vi "Teleop[Conflict 1].vi"(10 "Match Info":T3={"Autonomous Elapsed Seconds"=0.0, "TeleOp Elapsed Seconds"=0.0, "Disabled Elapsed Seconds"=0.0, "Visited Autonomous"=FALSE, "Visited TeleOp"=FALSE, "Visited Disabled"=FALSE, "Autonomous Settings"={"Autonomous Style"=enum."Independent", "VI Refnum"=refnum}}, 11 "Call Context":T4) -> ()   [LabVIEW 2019]
doc: "This VI is called for each TeleOp packet received from the DS where the robot is not disabled. It is often used to read from the joysticks and update I/O or to update setpoints for timed control loops. It should complete and return within 20 milliseconds or it may miss DS packets."
uses:
  <vilib>/Rock Robotics/WPI/DriverStation/WPI_DriverStationDerivedRobotMode.ctl
  <vilib>/Rock Robotics/WPI/DriverStation/WPI_DriverStationMatch Info.ctl
  <vilib>/Rock Robotics/WPI/ThirdParty/Phoenix-LabVIEW/Motor Controller/Controls/CTRE_Phoenix_MotorControl_ControlMode.ctl
  <vilib>/Rock Robotics/WPI/Utilities/WPI_GetSetVariantRefNum.vi
  <vilib>/Rock Robotics/WPI/Joystick/WPI_JoystickArcadeMapping.vi
  Toolbox/Piston/Piston Toggle.vi
  <vilib>/Rock Robotics/WPI/Solenoid/WPI_SolenoidSetEnum.vi
  <vilib>/Rock Robotics/Network Tables/NT Write Number.vi
  <vilib>/Rock Robotics/Network Tables/NT Read Number.vi
  <vilib>/addons/control/pid/pid.llb/PID (DBL).vi
  <vilib>/Rock Robotics/WPI/ThirdParty/Phoenix-LabVIEW/Motor Controller/Get/CTRE_Phoenix_MotorController_GetSupplyAndStatorCurrent_Enhanced.vi
  <vilib>/addons/control/pid/NI_PID_pid.lvlib
panel:
  in  "Magazine Power":dbl=0.25
  in  "Shooter Power":dbl=1.0
  in  "Magazine Overflow Power":dbl=-1.0
  in  "Magazine Intake Power":dbl=0.25
  in  "Intake power":dbl=0.7
  out "Shooter Motor Current":T1(graph)
  out "tx":dbl
  in  "PID gains":T2={"proportional gain (Kc)"=0.025, "integral time (Ti, min)"=0.01, "derivative time (Td, min)"=0.0} {"derivative time (Td, min)" format="%.3g"; "integral time (Ti, min)" format="%.3e"; "proportional gain (Kc)" format="%.3g"}
  in  "Winch Power":dbl=1.0
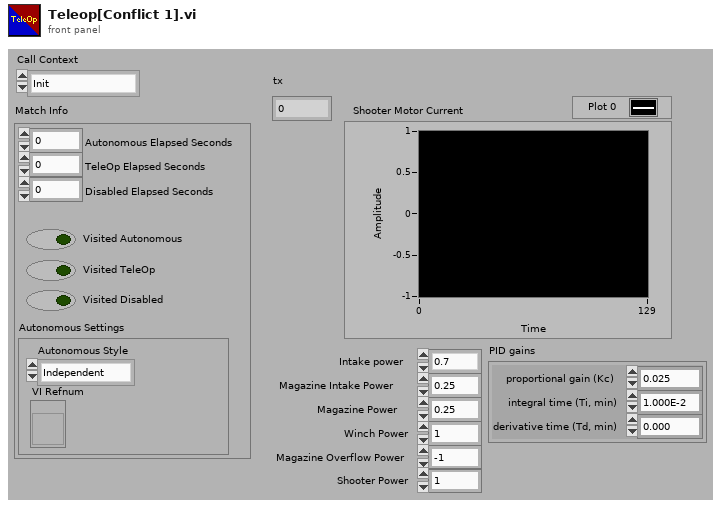
[diagram p1: front panel]
types:
  T1 = cluster{"Supply Current":dbl, "Stator Current":dbl}
  T2 = cluster{"proportional gain (Kc)":dbl, "integral time (Ti, min)":dbl, "derivative time (Td, min)":dbl}
  T3 = typedef "WPI_DriverStationMatch Info.ctl" = cluster{"Autonomous Elapsed Seconds":dbl, "TeleOp Elapsed Seconds":dbl, "Disabled Elapsed Seconds":dbl, "Visited Autonomous":bool, "Visited TeleOp":bool, "Visited Disabled":bool, "Autonomous Settings":cluster{"Autonomous Style":enum16{"Iterative", "Independent"}, "VI Refnum":refnum<vi>}}
  T4 = typedef "WPI_DriverStationDerivedRobotMode.ctl" = enum16{"Init", "Execute", "Stop"}
  T5 = typedef "CTRE_Phoenix_MotorControl_ControlMode.ctl" = u16
  T6 = cluster{"Intake In":bool, "Intake Out":bool, "Magazine In":bool, "Magazine Out":bool, "Winch In":bool, "Winch Out":bool, "Climber Hold":bool, "Intake Pistons":bool, "Shooter Hold":bool, "None":bool, "Power Toggle":bool, "Auto Target":bool}
  T7 = typedef "WPI_JoystickDevRef.ctl" = cluster{"Device":T8}
  T8 = typedef "WPI_JoystickDeviceEnum.ctl" = enum16{"USB 0", "USB 1", "USB 2", "USB 3", "USB 4", "USB 5"}
  T9 = typedef "WPI_MotorControlDeviceRef.ctl" = cluster{"DeviceStatus":errorcluster, "Type":T10, "PWM":cluster{"PWM Channel":T11, "DeadBand":T12}, "CAN":cluster{"Device Number":u8, "SetOutput VI Ref":variant, "GetOutput VI Ref":variant, "Enable VI Ref":variant, "Disable VI Ref":variant, "Data":variant}, "Invert":bool, "DIO PWM":cluster{"PWM \"Enable\" Channel":T11, "DIOChannel":T13, "PWM Rate":dbl}}
  T10 = typedef "WPI_MotorControlType.ctl" = enum16{"PWM", "CAN", "DIO PWM"}
  T11 = typedef "FPGA_DIOPWMChannel.ctl" = enum8{"PWM 0", "PWM 1", "PWM 2", "PWM 3", "PWM 4", "PWM 5", "PWM 6", "PWM 7", "PWM 8", "PWM 9", "PWM MXP 0", "PWM MXP 1", "PWM MXP 2", "PWM MXP 3", "PWM MXP 4", "PWM MXP 5", "PWM MXP 6", "PWM MXP 7", "PWM MXP 8", "PWM MXP 9", "Invalid"}
  T12 = typedef "WPI_PWMDeadband.ctl" = cluster{"Name":string, "maxPositivePwm":i32, "minPositivePwm":i32, "centerPwm":i32, "maxNegativePwm":i32, "minNegativePwm":i32, "angularRange":u16}
  T13 = typedef "FPGA_DIOChannel.ctl" = enum8{"DIO 0", "DIO 1", "DIO 2", "DIO 3", "DIO 4", "DIO 5", "DIO 6", "DIO 7", "DIO 8", "DIO 9", "DIO MXP 0", "DIO MXP 1", "DIO MXP 2", "DIO MXP 3", "DIO MXP 4", "DIO MXP 5", "DIO MXP 6", "DIO MXP 7", "DIO MXP 8", "DIO MXP 9", "DIO MXP 10", "DIO MXP 11", "DIO MXP 12", "DIO MXP 13", "DIO MXP 14", "DIO MXP 15", "SPI Port CS1", "SPI Port CS2", "SPI Port CS3", "SPI Port MISO", "SPI Port MOSI", "Invalid"}
  T14 = typedef "WPI_SolenoidValue.ctl" = enum16{"Off", "On", "Forward", "Reverse"}
  T15 = typedef "WPI_SolenoidDevRef.ctl" = cluster{"DevStatus":errorcluster, "Pneumatics Control Module":u8, "Forward Solenoid Channel":T16, "Reverse Solenoid Channel":T16}
  T16 = typedef "WPI_SolenoidChannel.ctl" = enum8{"Solenoid 0", "Solenoid 1", "Solenoid 2", "Solenoid 3", "Solenoid 4", "Solenoid 5", "Solenoid 6", "Solenoid 7", "Invalid"}
  T17 = typedef "WPI_DigitalInputDevRef.ctl" = cluster{"DevStatus":errorcluster, "DIO Channel":T13}
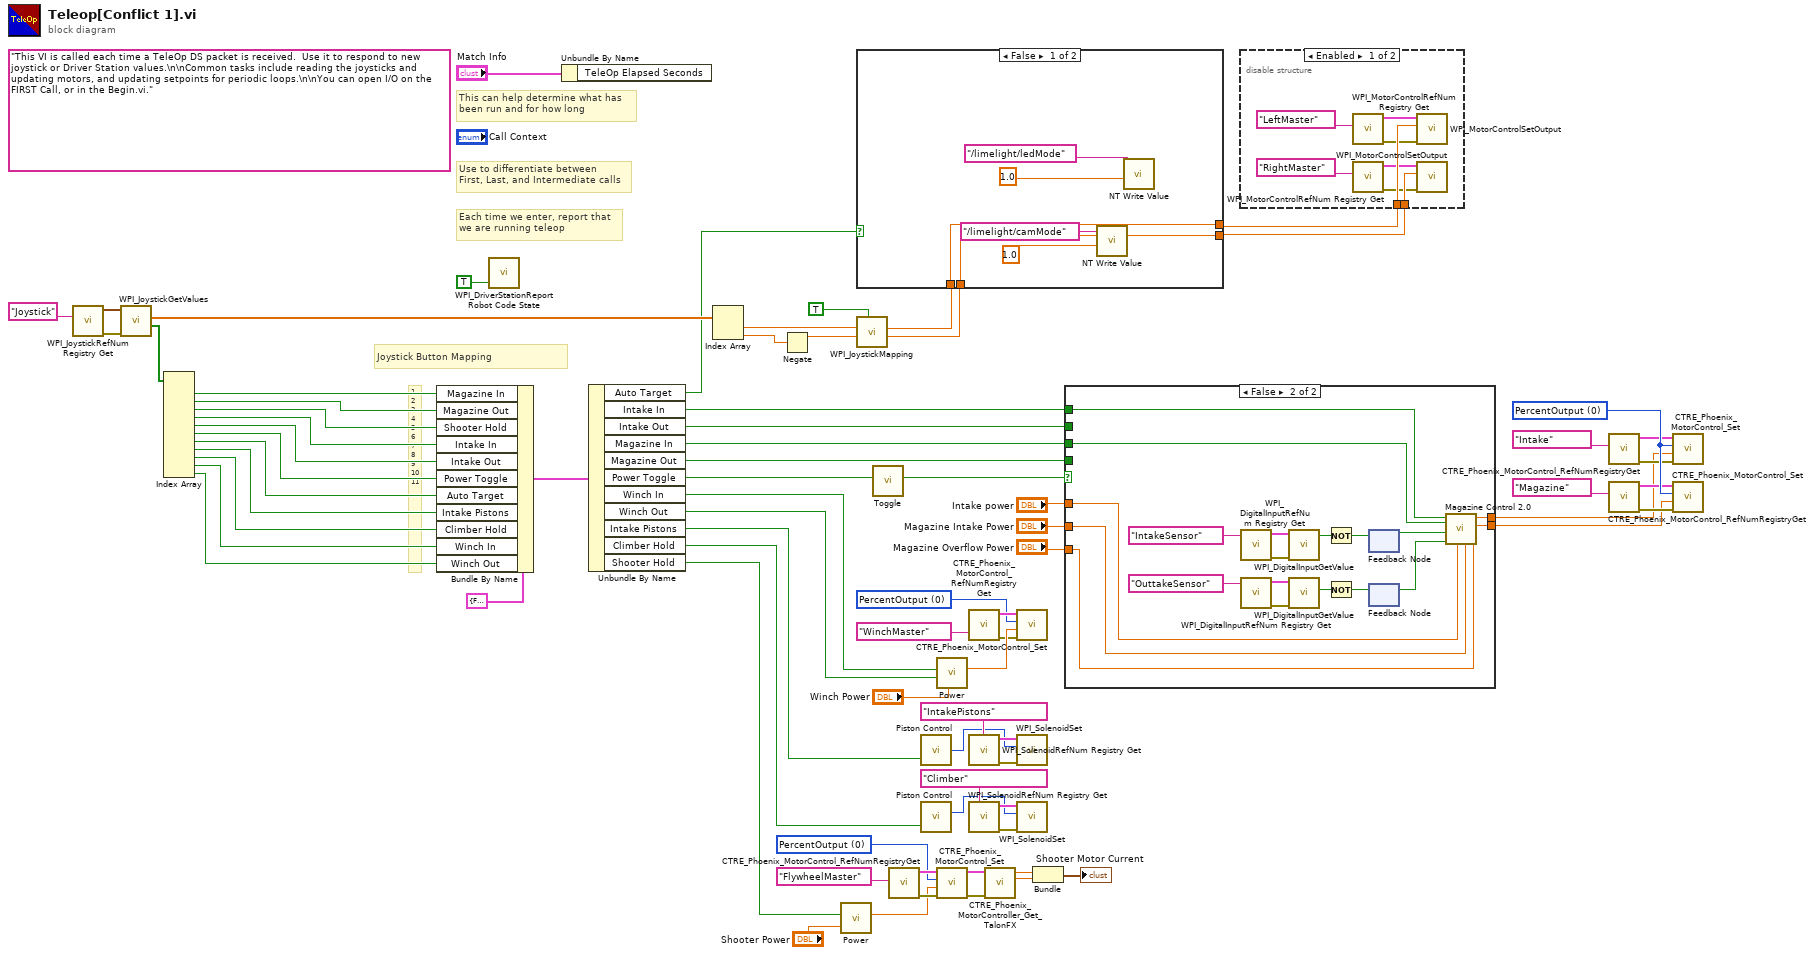
[diagram p0: block diagram]
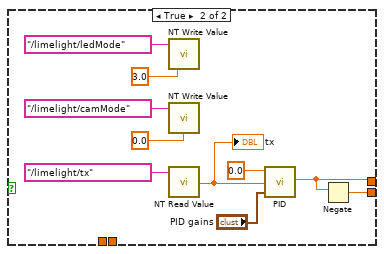
[diagram p2: hidden frame]
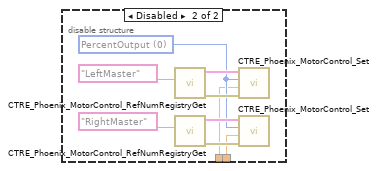
[diagram p3: hidden frame]
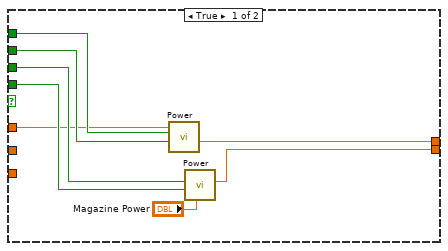
[diagram p4: hidden frame]
diagram:
  w8 = T5 0 items=["PercentOutput"=0, "Position"=1, "Velocity"=2, "Current"=3, "Follower"=5, "MotionProfile"=6, "MotionMagic"=7, "MotionProfileArc"=10, "Disabled"=15] ("Control Mode")
  w21 = T5 0 items=["PercentOutput"=0, "Position"=1, "Velocity"=2, "Current"=3, "Follower"=5, "MotionProfile"=6, "MotionMagic"=7, "MotionProfileArc"=10, "Disabled"=15] ("Control Mode")
  w25 = T5 0 items=["PercentOutput"=0, "Position"=1, "Velocity"=2, "Current"=3, "Follower"=5, "MotionProfile"=6, "MotionMagic"=7, "MotionProfileArc"=10, "Disabled"=15] ("Control Mode")
  (unwired) "This VI is called each time a TeleOp DS packet is received.  Use it to respond to new joystick or Driver Station values.\n\nCommon tasks include reading the joysticks and updating motors, and updating setpoints for periodic loops.\n\nYou can open I/O on the FIRST Call, or in the Begin.vi."
  # "1\n2\n3\n4\n5\n6\n7\n8\n9\n10\n11"
  # "Joystick Button Mapping"
  # "Each time we enter, report that\nwe are running teleop"
  # "Use to differentiate between\nFirst, Last, and Intermediate calls"
  # "This can help determine what has\nbeen run and for how long"
  n1 = call <vilib>:"WPI_JoystickRefNum Registry Get.vi"("refnum name"="Joystick") -> ("error out"=w75:errorcluster, "JoystickDevRef"=w74:T7)  [unwired: 9 in]
  n2 = call <vilib>:"WPI_JoystickGetValues.vi"("error in (no error)"=w75, "JoystickDevRef"=w74) -> ("Buttons"=w57:bool[], "Axes"=w72:dbl[])  [unwired: 5 in, 3 out]
  n3 = Index Array(array=w57) -> (element #1=w58:bool, element #2=w29:bool, element #3=w66:bool, element #4=w30:bool, element #5=w65:bool, element #6=w64:bool, element #7=w63:bool, element #8=w62:bool, element #9=w61:bool, element #10=w60:bool, element #11=w59:bool)  [unwired: 11 in]
  n4 = Bundle By Name(cluster=T6 {"Intake In"=FALSE, "Intake Out"=FALSE, "Magazine In"=FALSE, "Magazine Out"=FALSE, "Winch In"=FALSE, "Winch Out"=FALSE, "Climber Hold"=FALSE, "Intake Pistons"=FALSE, "Shooter Hold"=FALSE, "None"=FALSE, "Power Toggle"=FALSE, "Auto Target"=FALSE} ("input cluster"), "Magazine In"=w58, "Magazine Out"=w29, "Shooter Hold"=w66, "Intake In"=w30, "Intake Out"=w65, "Power Toggle"=w64, "Auto Target"=w63, "Intake Pistons"=w62, "Climber Hold"=w61, "Winch In"=w60, "Winch Out"=w59) -> (w56:T6)
  n5 = call <vilib>:"WPI_DriverStationReport Robot Code State.vi"("TeleOp"=TRUE ("Autonomous")) -> ()  [unwired: 10 in, 1 out]
  n6 = Unbundle By Name("Match Info") -> ()  [unwired: 1 out]
  n7 = Unbundle By Name(w56) -> ("Auto Target"=w39:bool, "Intake In"=w44:bool, "Intake Out"=w55:bool, "Magazine In"=w54:bool, "Magazine Out"=w53:bool, "Power Toggle"=w23:bool, "Winch In"=w52:bool, "Winch Out"=w51:bool, "Intake Pistons"=w36:bool, "Climber Hold"=w35:bool, "Shooter Hold"=w12:bool)
  n8 = Index Array(array=w72) -> (element #1=w71:dbl, element #2=w69:dbl)  [unwired: 2 in]
  n9 = Negate(x=w69) -> (-x=w70:dbl)
  n10 = call "Power.vi"("Positive Power"="Shooter Power", "Positive"=w12) -> ("Output"=w2:dbl)  [unwired: 9 in]
  n11 = call-poly <vilib>:"WPI_JoystickMapping.vi"("Square Inputs"=TRUE, "Y axis value"=w70, "X axis value"=w71) -> ("Right Motor Value"=w42:dbl, "Left Motor Value"=w43:dbl)  [unwired: 7 in]
  n12 = case shown="False" w39 {
    tunnel: w43 -> [w83 _]
    tunnel: w42 -> [w82 _]
    tunnel: [w83 w88] -> w41
    tunnel: [w82 w89] -> w40
    frame False {
      n13 = call-poly <vilib>:"NT Write Value.vi"("Numeric"=1.0, "Name"="/limelight/camMode") -> ()  [unwired: 9 in, 1 out]
      n14 = call-poly <vilib>:"NT Write Value.vi"("Numeric"=1.0, "Name"="/limelight/ledMode") -> ()  [unwired: 9 in, 1 out]
    }
    frame True {
      n15 = call-poly <vilib>:"NT Write Value.vi"("Numeric"=3.0, "Name"="/limelight/ledMode") -> ()  [unwired: 9 in, 1 out]
      n16 = call-poly <vilib>:"NT Write Value.vi"("Numeric"=0.0, "Name"="/limelight/camMode") -> ()  [unwired: 9 in, 1 out]
      n17 = call-poly <vilib>:"NT Read Value.vi"("Name"="/limelight/tx") -> ("Numeric"=w92:dbl)  [unwired: 9 in, 1 out]
      "tx" <- w92
      n18 = call-poly <vilib>:"PID.vi"("PID gains"="PID gains", "process variable"=w92, "setpoint"=0.0) -> ("output"=w88:dbl)  [unwired: 7 in, 1 out]
      n19 = Negate(x=w88) -> (-x=w89:dbl)
    }
  }
  n20 = call "Toggle.vi"("Input"=w23) -> ("Output"=w24:bool)  [unwired: 10 in]
  n21 = call <vilib>:"CTRE_Phoenix_MotorControl_RefNumRegistryGet.vi"("refnum name"="FlywheelMaster") -> ("error out"=w10:errorcluster, "PhoenixMotorControlDevRef"=w9:T9)  [unwired: 9 in]
  n22 = call-poly "Piston Control.vi"("Input"=w36) -> ("Output"=w38:T14)  [unwired: 1 in]
  n23 = call-poly "Piston Control.vi"("Input"=w35) -> ("Output"=w37:T14)  [unwired: 1 in]
  n24 = call "Power.vi"("Positive Power"="Winch Power", "Negative"=w51, "Positive"=w52) -> ("Output"=w67:dbl)  [unwired: 8 in]
  n25 = call <vilib>:"CTRE_Phoenix_MotorControl_Set.vi"("error in (no error)"=w10, "Output"=w2, "Control Mode"=w8, "PhoenixMotorControlDevRef"=w9) -> ("error out"=w6:errorcluster, "PhoenixMotorControlDevRef"=w7:T9)  [unwired: 6 in]
  n26 = call <vilib>:"CTRE_Phoenix_MotorControl_RefNumRegistryGet.vi"("refnum name"="WinchMaster") -> ("error out"=w27:errorcluster, "PhoenixMotorControlDevRef"=w26:T9)  [unwired: 9 in]
  n27 = call <vilib>:"WPI_SolenoidRefNum Registry Get.vi"("refnum name"="IntakePistons") -> ("error out"=w50:errorcluster, "SolenoidDevRef"=w49:T15)  [unwired: 9 in]
  n28 = call <vilib>:"WPI_SolenoidRefNum Registry Get.vi"("refnum name"="Climber") -> ("error out"=w47:errorcluster, "SolenoidDevRef"=w46:T15)  [unwired: 9 in]
  n29 = call-poly <vilib>:"CTRE_Phoenix_MotorController_Get_TalonFX.vi"("PhoenixMotorControlDevRef"=w7, "error in"=w6) -> ("Supply Current"=w5:dbl, "Stator Current"=w4:dbl)  [unwired: 10 in, 2 out]
  n30 = call <vilib>:"CTRE_Phoenix_MotorControl_Set.vi"("error in (no error)"=w27, "Output"=w67, "Control Mode"=w25, "PhoenixMotorControlDevRef"=w26) -> ()  [unwired: 6 in, 2 out]
  n31 = call-poly <vilib>:"WPI_SolenoidSet.vi"("error in (no error)"=w50, "Value"=w38, "SolenoidDevRef"=w49) -> ()  [unwired: 7 in, 2 out]
  n32 = call-poly <vilib>:"WPI_SolenoidSet.vi"("error in (no error)"=w47, "Value"=w37, "SolenoidDevRef"=w46) -> ()  [unwired: 7 in, 2 out]
  n33 = Bundle("Supply Current"=w5, "Stator Current"=w4) -> (→"Shooter Motor Current":T1)  [unwired: 1 in]
  n34 = case shown="False" w24 {
    tunnel: w55 -> [w101 _]
    tunnel: w54 -> [w100 w107]
    tunnel: w53 -> [w99 _]
    tunnel: w44 -> [w98 w110]
    tunnel: [w96 w103] -> w14
    tunnel: [w97 w102] -> w13
    tunnel: "Magazine Overflow Power" -> [_ w104]
    tunnel: "Magazine Intake Power" -> [_ w105]
    tunnel: "Intake power" -> [w95 w106]
    frame True {
      n35 = call "Power.vi"("Positive Power"=w95, "Negative"=w101, "Positive"=w98) -> ("Output"=w96:dbl)  [unwired: 8 in]
      n36 = call "Power.vi"("Positive Power"="Magazine Power", "Negative"=w99, "Positive"=w100) -> ("Output"=w97:dbl)  [unwired: 8 in]
    }
    frame False {
      n37 = call <vilib>:"WPI_DigitalInputRefNum Registry Get.vi"("refnum name"="IntakeSensor") -> ("error out"=w120:errorcluster, "DigitalInputDevRef"=w119:T17)  [unwired: 9 in]
      n38 = call <vilib>:"WPI_DigitalInputRefNum Registry Get.vi"("refnum name"="OuttakeSensor") -> ("error out"=w117:errorcluster, "DigitalInputDevRef"=w118:T17)  [unwired: 9 in]
      n39 = call <vilib>:"WPI_DigitalInputGetValue.vi"("error in (no error)"=w120, "DigitalInputDevRef"=w119) -> ("Value"=w116:bool)  [unwired: 7 in, 2 out]
      n40 = call <vilib>:"WPI_DigitalInputGetValue.vi"("error in (no error)"=w117, "DigitalInputDevRef"=w118) -> ("Value"=w115:bool)  [unwired: 7 in, 2 out]
      n41 = Not(x=w116) -> (.not. x?=w112:bool)
      n42 = Not(x=w115) -> (.not. x?=w111:bool)
      n43 = feedback-in #1(w112) -> ()
      n44 = feedback #1() -> (w108:bool)  [unwired: 1 in]
      n45 = feedback #2() -> (w109:bool)  [unwired: 1 in]
      n46 = feedback-in #2(w111) -> ()
      n47 = call "Magazine Control 2.0.vi"("Magazine Overflow Power"=w104, "Magazine Power"=w105, "Intake Power"=w106, "Outtake Sensor"=w109, "Intake Sensor"=w108, "Outtake Button"=w107, "Intake Button"=w110) -> ("Magazine"=w102:dbl, "Intake"=w103:dbl)  [unwired: 3 in]
    }
  }
  n48 = disable-structure shown="Enabled" {
    disable-tunnel: w41 -> [w128 w130]
    disable-tunnel: w40 -> [w127 w129]
    frame Enabled {
      n49 = call <vilib>:"WPI_MotorControlRefNum Registry Get.vi"("refnum name"="LeftMaster") -> ("error out"=w124:errorcluster, "MotorControlDevRef"=w123:T9)  [unwired: 9 in]
      n50 = call <vilib>:"WPI_MotorControlRefNum Registry Get.vi"("refnum name"="RightMaster") -> ("error out"=w122:errorcluster, "MotorControlDevRef"=w121:T9)  [unwired: 9 in]
      n51 = call <vilib>:"WPI_MotorControlSetOutput.vi"("error in (no error)"=w124, "Output"=w128, "MotorControlDevRef"=w123) -> ()  [unwired: 6 in, 3 out]
      n52 = call <vilib>:"WPI_MotorControlSetOutput.vi"("error in (no error)"=w122, "Output"=w127, "MotorControlDevRef"=w121) -> ()  [unwired: 6 in, 3 out]
    }
    frame Disabled {
      w131 = T5 0 items=["PercentOutput"=0, "Position"=1, "Velocity"=2, "Current"=3, "Follower"=5, "MotionProfile"=6, "MotionMagic"=7, "MotionProfileArc"=10, "Disabled"=15] ("Control Mode")
      n53 = call <vilib>:"CTRE_Phoenix_MotorControl_RefNumRegistryGet.vi"("refnum name"="LeftMaster") -> ("error out"=w135:errorcluster, "PhoenixMotorControlDevRef"=w134:T9)  [unwired: 9 in]
      n54 = call <vilib>:"CTRE_Phoenix_MotorControl_RefNumRegistryGet.vi"("refnum name"="RightMaster") -> ("error out"=w133:errorcluster, "PhoenixMotorControlDevRef"=w132:T9)  [unwired: 9 in]
      n55 = call <vilib>:"CTRE_Phoenix_MotorControl_Set.vi"("error in (no error)"=w135, "Output"=w130, "Control Mode"=w131, "PhoenixMotorControlDevRef"=w134) -> ()  [unwired: 6 in, 2 out]
      n56 = call <vilib>:"CTRE_Phoenix_MotorControl_Set.vi"("error in (no error)"=w133, "Output"=w129, "Control Mode"=w131, "PhoenixMotorControlDevRef"=w132) -> ()  [unwired: 6 in, 2 out]
    }
  }
  n57 = call <vilib>:"CTRE_Phoenix_MotorControl_RefNumRegistryGet.vi"("refnum name"="Intake") -> ("error out"=w17:errorcluster, "PhoenixMotorControlDevRef"=w18:T9)  [unwired: 9 in]
  n58 = call <vilib>:"CTRE_Phoenix_MotorControl_RefNumRegistryGet.vi"("refnum name"="Magazine") -> ("error out"=w19:errorcluster, "PhoenixMotorControlDevRef"=w20:T9)  [unwired: 9 in]
  n59 = call <vilib>:"CTRE_Phoenix_MotorControl_Set.vi"("error in (no error)"=w17, "Output"=w14, "Control Mode"=w21, "PhoenixMotorControlDevRef"=w18) -> ()  [unwired: 6 in, 2 out]
  n60 = call <vilib>:"CTRE_Phoenix_MotorControl_Set.vi"("error in (no error)"=w19, "Output"=w13, "Control Mode"=w21, "PhoenixMotorControlDevRef"=w20) -> ()  [unwired: 6 in, 2 out]
